vi "Terminate.vi"(8 "error in (no error)":errorcluster, 10 "Message in":refnum<class "TerminateMessage.lvclass">, 11 "Tomo in":refnum<class "Tomo.lvclass">) -> (0 "error out":errorcluster, 3 "Tomo out":refnum<class "Tomo.lvclass">)   [LabVIEW 2012, in "Tomo.lvclass"]
doc: "This member function is called when the statemachine in the run.vi receives an 'terminate' command. It closes the RabbitMQ connection. \n\nOverride this member function in your derived class to release all previously acquired resources (but don't forget to call the parent method). If your component has subcomponents, they count as resources, and you have to release them by calling their own terminate functions."
uses:
  Tomo.lvclass
  <vilib>/Distrio/Murmex/TerminateMessage/TerminateMessage.lvclass
  <vilib>/Distrio/Murmex/Murmex/Murmex.lvclass
  Tomo.lvclass/Tomo.ctl
panel:
  # "This method is called when the TERMINATE\ntrigger is sent. \n\nOverride this method when your component needs to\nrespond to this trigger. \n\nCall parent for proper implementation"
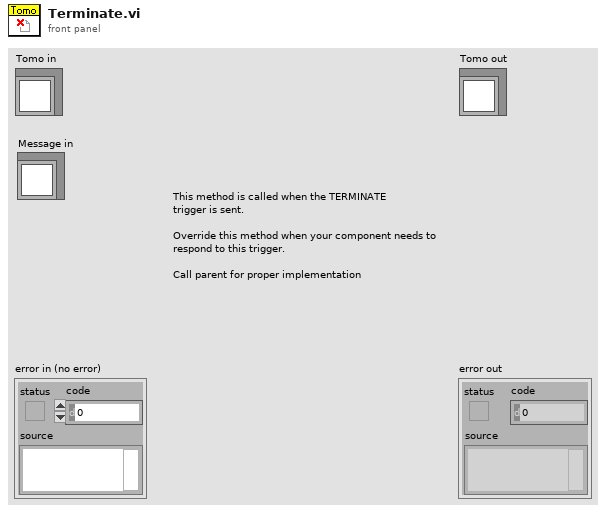
[diagram p1: front panel]
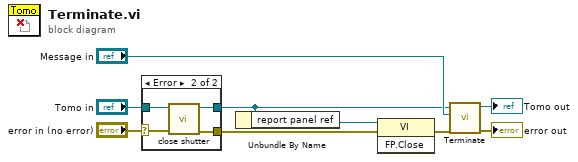
[diagram p0: block diagram]
diagram:
  n1 = case shown="Error" "error in (no error)" {
    selector: "error in (no error)" -> [w10 w15]
    tunnel: [w10 w14] -> w1
    tunnel: "Tomo in" -> [w11 w13]
    tunnel: [w11 w12] -> w4
    frame No Error {
    }
    frame Error {
      n2 = call "close shutter.vi"("error in (no error)"=w15, "Murmex in"=w13) -> ("error out"=w14:errorcluster, "Murmex out"=w12:refnum<class "Tomo.lvclass">)  [unwired: 8 in]
    }
  }
  n3 = Unbundle By Name(w4) -> ("report panel ref"=w3:refnum<vi>)
  n4 = invoke class="VI" method="FP.Close"(reference=w3, error in=w1) -> (error out=w2:errorcluster)  [unwired: 1 in, 2 out]
  n5 = call-parent "Terminate.vi"("error in (no error)"=w2, "Message in"="Message in", "Murmex in"=w4) -> ("error out"=→"error out":errorcluster, "Murmex out"=→"Tomo out":refnum<class "Tomo.lvclass">)  [unwired: 7 in]
